vi "Print Variable.vi"(8 "error in (no error)":errorcluster, 9 "Variable Name":string, 10 "Variable Type (0: Number)":i32(ring) items=["Number", "Message"], 11 "VISA resource name":refnum<visa-resource-name>) -> (0 "error out":errorcluster, 1 "Message":string, 2 "Number":dbl, 3 "VISA resource name out":refnum<visa-resource-name>)   [LabVIEW 2019, in "Keithley 2600 Series.lvlib"]
doc: "Prints the variable data.\n\n<b>Note:</b>\nWhen you run a script that contains the command of \"print()\", you need to call this VI and set the variable name to \"Nil\" to read the output data or message."
uses:
  <instrlib>/Keithley 2600 Series/Keithley 2600 Series.lvlib
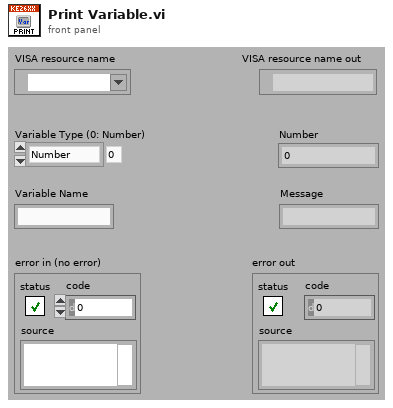
[diagram p1: front panel]
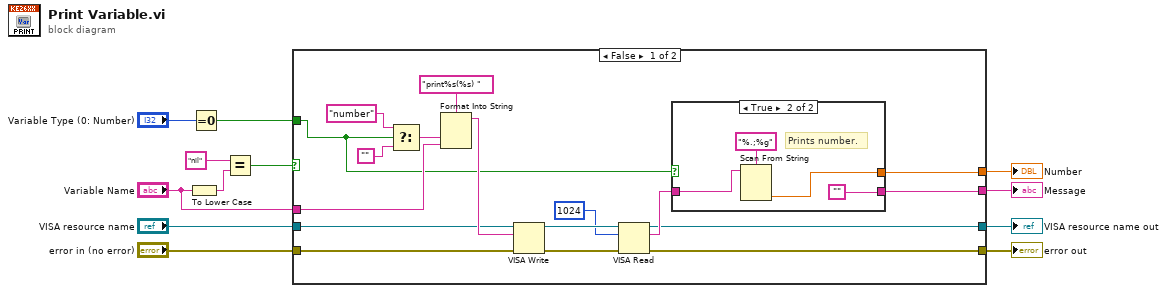
[diagram p0: block diagram]
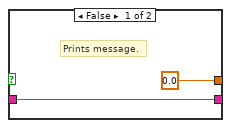
[diagram p2: hidden frame]
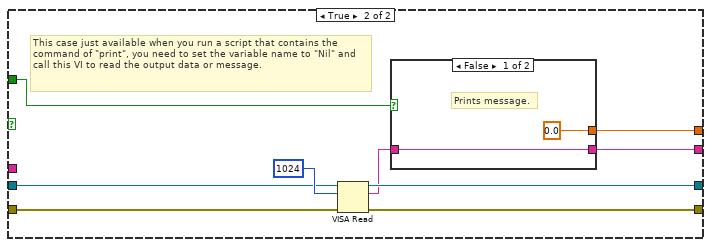
[diagram p3: hidden frame]
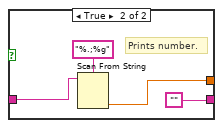
[diagram p4: hidden frame]
diagram:
  n1 = To Lower Case(string="Variable Name") -> (all lower case string=w8:string)
  n2 = Equal To 0?(x="Variable Type (0: Number)") -> (x = 0?=w11:bool)
  n3 = Equal?(x="nil", y=w8) -> (x = y?=w6:bool)
  n4 = case shown="False" w6 {
    tunnel: [w14 w44] -> w2
    tunnel: [w13 w43] -> w1
    tunnel: w11 -> [w15 w41]
    tunnel: [w16 w39] -> w10
    tunnel: [w17 w38] -> w9
    tunnel: "VISA resource name" -> [w20 w37]
    tunnel: "error in (no error)" -> [w18 w36]
    tunnel: "Variable Name" -> [w19 _]
    frame False {
      n5 = Select(t="number", s=w15, f="") -> (s? t:f=w27:string)
      n6 = Format Into String(format string="print%s(%s) ", w27, w19) -> (resulting string=w26:string)  [unwired: 2 in, 1 out]
      n7 = VISA Write(VISA resource name=w20, write buffer=w26, error in (no error)=w18) -> (VISA resource name out=w25:refnum<visa-resource-name>, error out=w24:errorcluster)  [unwired: 1 out]
      n8 = VISA Read(VISA resource name=w25, byte count=u32 1024, error in (no error)=w24) -> (VISA resource name out=w14:refnum<visa-resource-name>, read buffer=w22:string, error out=w13:errorcluster)  [unwired: 1 out]
      n9 = case shown="True" w15 {
        tunnel: w22 -> [w31 w34]
        tunnel: [w31 ""] -> w16
        tunnel: [0.0 w32] -> w17
        frame False {
          # "Prints message."
        }
        frame True {
          # "Prints number."
          n10 = Scan From String(format string="%.;%g", input string=w34) -> (output 1=w32:dbl)  [unwired: 3 in, 3 out]
        }
      }
    }
    frame True {
      # "This case just available when you run a script that contains the command of \"print\", you need to set the variable name to \"Nil\" and call this VI to read the output data or message."
      n11 = VISA Read(VISA resource name=w37, byte count=u32 1024, error in (no error)=w36) -> (VISA resource name out=w44:refnum<visa-resource-name>, read buffer=w40:string, error out=w43:errorcluster)  [unwired: 1 out]
      n12 = case shown="False" w41 {
        tunnel: w40 -> [w46 w49]
        tunnel: [w46 ""] -> w39
        tunnel: [0.0 w47] -> w38
        frame False {
          # "Prints message."
        }
        frame True {
          # "Prints number."
          n13 = Scan From String(format string="%.;%g", input string=w49) -> (output 1=w47:dbl)  [unwired: 3 in, 3 out]
        }
      }
    }
  }
  "VISA resource name out" <- w2
  "error out" <- w1
  "Message" <- w10
  "Number" <- w9
